vi "Chirp.vi"(6 "Chirp/Fft Pair 1 - Chirp Rate":fxp<+/-,64,32>, 9 "Imaginary In":fxp<+/-,64,32>[](array[numeric])=[0.0, 0.0, 0.0, 0.0, 0.0, 0.0, 0.0, 0.0], 10 "Real In":fxp<+/-,64,32>[](array[numeric])=[0.0, 0.0, 0.0, 0.0, 0.0, 0.0, 0.0, 0.0]) -> (1 "Chirped Imaginary Out":fxp<+/-,64,32>[](array[numeric]), 2 "Chirped Real Out":fxp<+/-,64,32>[](array[numeric]))   [LabVIEW 2012]
panel:
  out "time":fxp<+/-,64,32>=26.843456943752244
  out "ang":fxp<+/-,64,32>=1.997984756482765
  out "c":fxp<+/-,32,16>=0.9999237060546875
  out "d":fxp<+/-,32,16>=-0.012664794921875
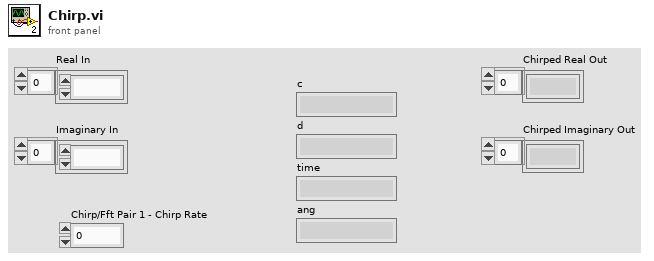
[diagram p1: front panel]
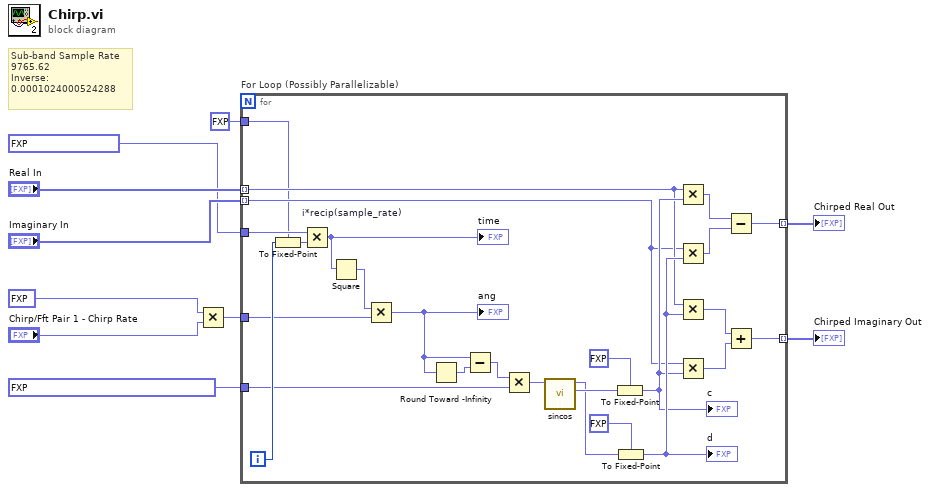
[diagram p0: block diagram]
diagram:
  # "Sub-band Sample Rate\n9765.62\nInverse:\n0.0001024000524288"
  n1 = Multiply(x=fxp<+/-,2,1> 0.5 ("Numeric"), y="Chirp/Fft Pair 1 - Chirp Rate") -> (x*y=w1:fxp<+/-,64,33>)
  n2 = for "For Loop (Possibly Parallelizable)" {
    tunnel: fxp<+,45,-13> 0.0001024000524287999 ("1/x") -> [w36]
    tunnel: "Real In" -> [w25] mode=indexing
    tunnel: "Imaginary In" -> [w24] mode=indexing
    tunnel: [w23] -> w8 mode=indexing
    tunnel: [w22] -> w7 mode=indexing
    tunnel: fxp<+/-,64,32> 0.0 ("Real In") -> [w21]
    tunnel: fxp<+/-,64,32> 6.283185307169333 ("Numeric") -> [w18]
    tunnel: w1 -> [w14]
    i -> [w35]
    n3 = To Fixed-Point(fixed-point type=w21, number=w35) -> (fixed-point=w34:fxp<+/-,64,32>)
    n4 = Multiply "i*recip(sample_rate)"(x=w36, y=w34) -> (x*y=w17:fxp<+/-,64,19>)
    "time" <- w17
    n5 = Square(x=w17) -> (x^2=w15:fxp<+,64,37>)
    n6 = Multiply(x=w15, y=w14) -> (x*y=w16:fxp<+/-,64,70>)
    "ang" <- w16
    n7 = Round Toward -Infinity(1:w16) -> (0:w33:fxp<+/-,64,70>)
    n8 = Subtract(x=w16, y=w33) -> (x-y=w32:fxp<+/-,64,71>)
    n9 = Multiply(x=w32, y=w18) -> (x*y=w13:fxp<+/-,64,103>)
    n10 = call "sincos.vi"("x (pi)"=w13) -> ("cos(x)"=w12:fxp<+/-,16,2>, "sin(x)"=w11:fxp<+/-,16,2>)  [unwired: 9 in]
    n11 = To Fixed-Point(fixed-point type=fxp<+/-,64,32> 0.0 ("Real In"), number=w12) -> (fixed-point=w26:fxp<+/-,64,32>)
    "c" <- w26
    n12 = To Fixed-Point(fixed-point type=fxp<+/-,64,32> 0.0 ("Real In"), number=w11) -> (fixed-point=w27:fxp<+/-,64,32>)
    "d" <- w27
    n13 = Multiply(x=w25, y=w26) -> (x*y=w31:fxp<+/-,64,64>)
    n14 = Multiply(x=w24, y=w27) -> (x*y=w30:fxp<+/-,64,64>)
    n15 = Multiply(x=w25, y=w27) -> (x*y=w28:fxp<+/-,64,64>)
    n16 = Multiply(x=w24, y=w26) -> (x*y=w29:fxp<+/-,64,64>)
    n17 = Subtract(x=w31, y=w30) -> (x-y=w23:fxp<+/-,64,65>)
    n18 = Add(x=w28, y=w29) -> (x+y=w22:fxp<+/-,64,65>)
  }
  "Chirped Real Out" <- w8
  "Chirped Imaginary Out" <- w7
